vi "main.vi"() -> ()   [LabVIEW 2017]
uses:
  main.Action.ctl
  PendulumLoop/PendulumLoop.Outputs.ci.vi
  PendulumLoop/PendulumLoop.lvlib
panel:
  in  "Set Force Zero":bool
  out "Cart Position":dbl(slide)=1.0 scale=-150.0..150.0
  out "Angle":dbl(knob) caption="Gauge"
  in  "Reset Camera":bool
  in  "Force":dbl(slide)=1.0 scale=-1000.0..1000.0
  in  "Simulation Data":T1={"plenght"=50.0, "cartMass"=10.0, "pendulumMass"=10.0, "angle"=0.0}
  in  "Reset Pendulum":bool
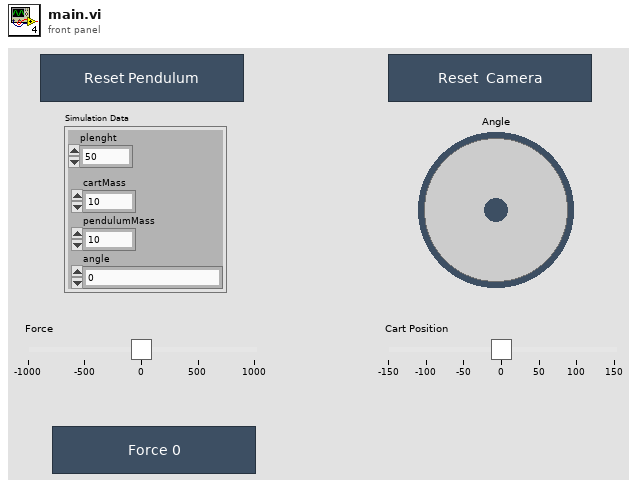
[diagram p1: front panel]
types:
  T1 = cluster{"plenght":dbl, "cartMass":dbl, "pendulumMass":dbl, "angle":dbl}
  T2 = typedef "main.Action.ctl" = enum16{"Init", "Wait for events", "Exit"}
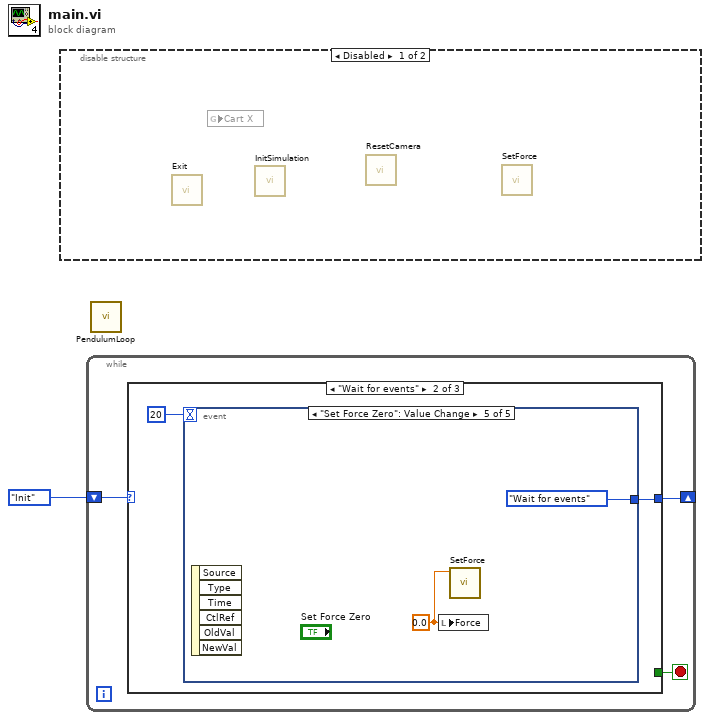
[diagram p0: block diagram]
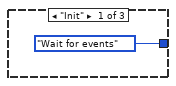
[diagram p2: hidden frame]
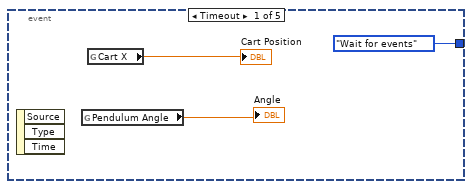
[diagram p3: hidden frame]
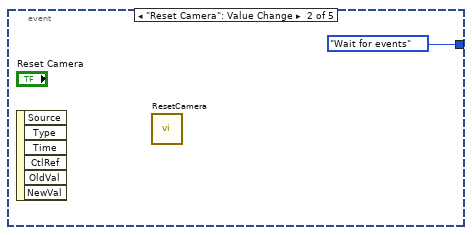
[diagram p4: hidden frame]
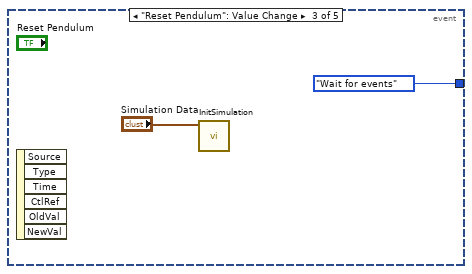
[diagram p5: hidden frame]
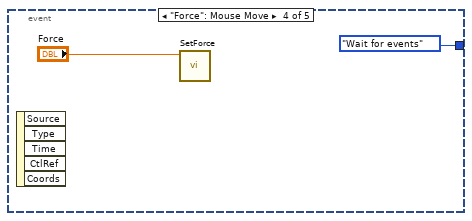
[diagram p6: hidden frame]
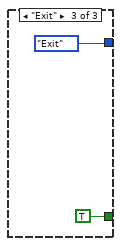
[diagram p7: hidden frame]
diagram:
  n1 = disable-structure shown="Disabled" {
    frame Disabled {
      n2 = call "Exit.vi"() -> ()  [unwired: 11 in, 1 out]
      n3 = global read "PendulumLoop.Outputs.ci.vi" "Cart X"() -> ()  [unwired: 1 in]
      n4 = call "InitSimulation.vi"() -> ()  [unwired: 11 in, 1 out]
      n5 = call "ResetCamera.vi"() -> ()  [unwired: 11 in, 1 out]
      n6 = call "SetForce.vi"() -> ()  [unwired: 11 in, 1 out]
    }
    frame Enabled {
    }
  }
  n7 = while {
    shift-right: [w3] -> _
    shift-left: main.Action."Init" -> [w4]
    stop <- w2 stop-if-true
    n8 = case shown="\"Wait for events\"" w4 {
      tunnel: [main.Action."Wait for events" w7 main.Action."Exit"] -> w3
      tunnel: [_ _ TRUE] -> w2
      frame "Init" {
      }
      frame "Wait for events" {
        n9 = event shown="[4] \"Set Force Zero\": Value Change" {
          selector: _ -> [_ _ _ _ _]
          dyn-events: _ -> [_ _ _ _ _]
          timeout: 20 -> [_ _ _ _ _]
          tunnel: [main.Action."Wait for events" main.Action."Wait for events" main.Action."Wait for events" main.Action."Wait for events" main.Action."Wait for events"] -> w7
          event Timeout {
            n10 = event-data() -> ()  [unwired: 1 in, 3 out]
            n11 = global read "PendulumLoop.Outputs.ci.vi" "Pendulum Angle"() -> (→"Angle":dbl)
            n12 = global read "PendulumLoop.Outputs.ci.vi" "Cart X"() -> (→"Cart Position":dbl)
          }
          event "Reset Camera": Value Change {
            n13 = event-data() -> ()  [unwired: 1 in, 6 out]
            n14 = call "ResetCamera.vi"() -> ()  [unwired: 11 in, 1 out]
          }
          event "Reset Pendulum": Value Change {
            n15 = event-data() -> ()  [unwired: 1 in, 6 out]
            n16 = call "InitSimulation.vi"("Simulation Data"="Simulation Data") -> ()  [unwired: 10 in, 1 out]
          }
          event "Force": Mouse Move {
            n17 = event-data() -> ()  [unwired: 1 in, 5 out]
            n18 = call "SetForce.vi"("Cart Force"="Force") -> ()  [unwired: 10 in, 1 out]
          }
          event "Set Force Zero": Value Change {
            w17 = 0.0 ("Force")
            n19 = event-data() -> ()  [unwired: 1 in, 6 out]
            n20 = local write "Force"(w17) -> ()
            n21 = call "SetForce.vi"("Cart Force"=w17) -> ()  [unwired: 10 in, 1 out]
          }
        }
      }
      frame "Exit" {
      }
    }
  }
  n22 = call "PendulumLoop.vi"() -> ()  [unwired: 12 in]
